vi "PUBLIC.constructor.vi"(0 "name":string, 2 "data in":string, 5 "error in (no error)":errorcluster) -> (14 "i ref out":refnum<vi>, 16 "data out":string, 19 "error out":errorcluster)   [LabVIEW 2014, in "KE6485GUI.lvlib"]
doc: "This is the constructor of a class.\n\nLicense Agreement for this software:\n\nCopyright (C)\nGesellschaft für Schwerionenforschung, GSI\nPlanckstr. 1\n64291 Darmstadt\nGermany\n\nContact: D.Beck@gsi.de \n\nThis program is free software; you can redistribute it and/or modify it under the terms of the \nGNU General Public License as published by the Free Software Foundation; either version 2 of \nthe license, or (at your option) any later version.\n\nThis program is distributed in the hope that it will be useful, but WITHOUT ANY WARRANTY; \nwithout even the implied warranty of MERCHANTABILITY or FITNESS FOR A PARTICULAR PURPOSE. See the GNU General License for more details (http://www.gnu.org).\n\nGesellschaft für Schwerionenforschung, GSI\nPlanckstr. 1, 64291 Darmstadt, Germany\nFor all questions and ideas contact: M.Richter@gsi.de, H.Brand@gsi.de or D.Beck@gsi.de.\nLast update: 16-JUN-2004"
uses:
  KE6485GUI.lvlib
  CSCore/CSObj/CSObj.lvlib
  CSCore/CSSystem/CSSystemLib/CSSystemLib.lvlib
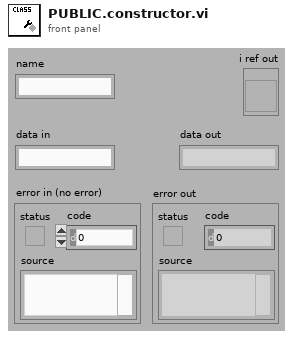
[diagram p1: front panel]
types:
  T1 = enum16{"SetAttribute", "GetAttribute", "CreateAttribute", "DestroyAttribute", "DestroyAllAtributes"}
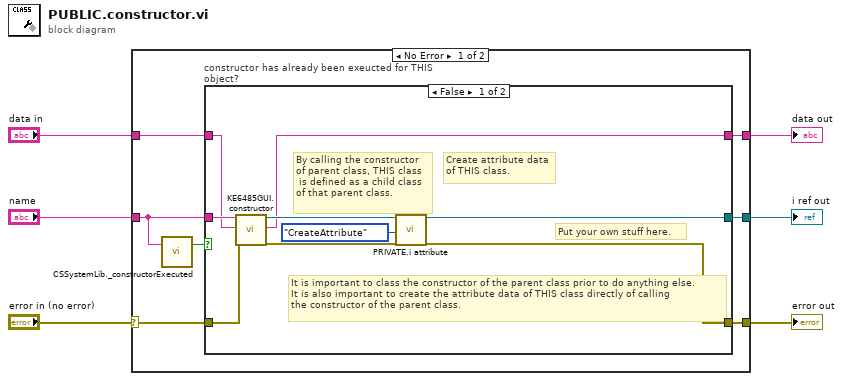
[diagram p0: block diagram]
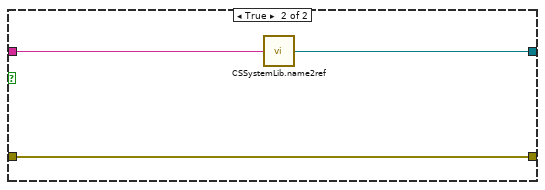
[diagram p2: hidden frame]
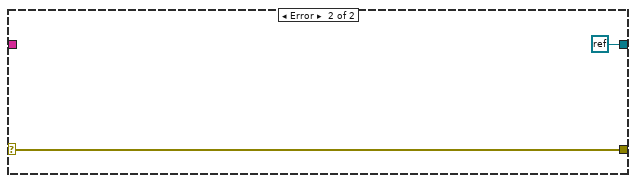
[diagram p3: hidden frame]
diagram:
  n1 = case shown="No Error" "error in (no error)" {
    selector: "error in (no error)" -> [w10 w26]
    tunnel: [w13 refnum<k0> refnum] -> w6
    tunnel: [w12 w26] -> w5
    tunnel: "name" -> [w8 _]
    tunnel: "data in" -> [w11 _]
    tunnel: [w7 _] -> w1
    frame No Error {
      n2 = call "CSSystemLib._constructorExecuted.vi"("name"=w8) -> ("constructor executed?"=w9:bool)  [unwired: 18 in]
      n3 = case "constructor has already been exeucted for THIS object?" shown="False" w9 {
        tunnel: [w19 w24] -> w13
        tunnel: [w18 w23] -> w12
        tunnel: w8 -> [w17 w25]
        tunnel: w11 -> [w16 _]
        tunnel: w10 -> [w15 w23]
        tunnel: [w14 _] -> w7
        frame False {
          # "It is important to class the constructor of the parent class prior to do anything else.\nIt is also important to create the attribute data of THIS class directly of calling\nthe constructor of the parent class."
          # "Put your own stuff here."
          # "Create attribute data\nof THIS class."
          # "By calling the constructor\nof parent class, THIS class\n is defined as a child class\nof that parent class."
          n4 = call "KE6485GUI.constructor.vi"("name"=w17, "data in"=w16, "error in (no error)"=w15) -> ("i ref out"=w22:refnum<vi>, "data out"=w14:string, "error out"=w21:errorcluster)  [unwired: 14 in]
          n5 = call "PRIVATE.i attribute.vi"("VI Refnum"=w22, "Action"=T1."CreateAttribute", "error in (no error)"=w21) -> ("VI Refnum out"=w19:refnum<vi>, "error out"=w18:errorcluster)  [unwired: 14 in, 1 out]
        }
        frame True {
          n6 = call "CSSystemLib.name2ref.vi"("name"=w25) -> ("obj refnum"=w24:refnum<vi>)
        }
      }
    }
    frame Error {
    }
  }
  "i ref out" <- w6
  "error out" <- w5
  "data out" <- w1
